vi "subGenPhaseContSine.vi"(0 "amplitude":dbl=1.0 format="%0.2p", 2 "reset signal":bool, 5 "frequency":dbl=10.0 format="%0.2p", 7 "phase":dbl format="%.2p", 11 "error in (no error)":errorcluster, 13 "sampling info":cluster{"Fs":dbl, "#s":dbl}={"Fs"=50000.0, "#s"=4000.0} {"Fs" format="%.2p"}) -> (4 "data":cluster{"t0":dbl, "dt":dbl, "Y":cdb[]}={"t0"=0.0, "dt"=1.0, "Y"=[]} {"Y" format="%.3f"; "dt" format="%^.2e"; "t0" format="%.4f"}, 8 "phase out":ext, 15 "error out":errorcluster)   [LabVIEW 2013]
uses:
  <vilib>/Analysis/1siggen.llb/Ramp Pattern by Samples.vi
  <vilib>/Analysis/NI_AALBase.lvlib
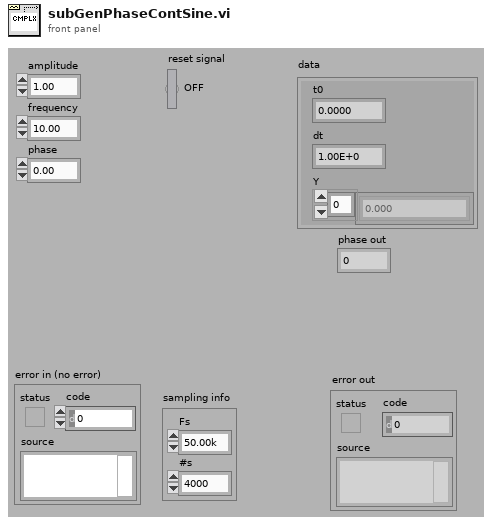
[diagram p1: front panel]
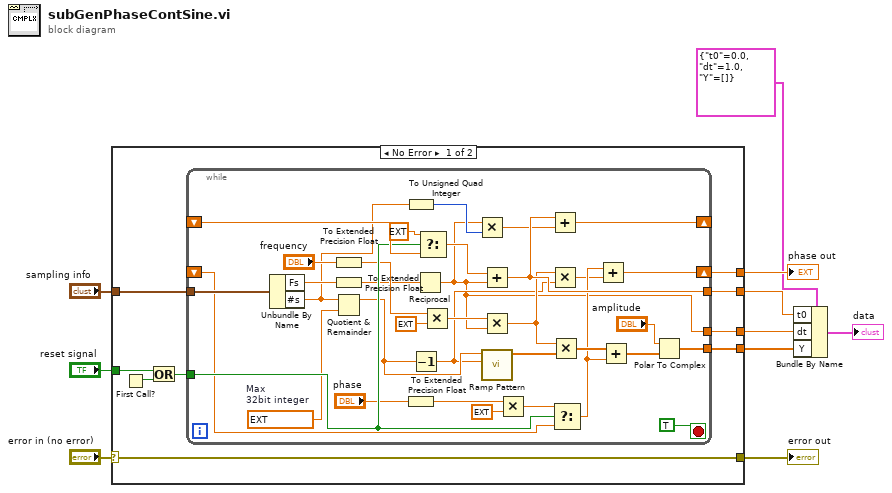
[diagram p0: block diagram]
diagram:
  n1 = case shown="No Error" "error in (no error)" {
    selector: "error in (no error)" -> [w11 w55]
    tunnel: "sampling info" -> [w19 _]
    tunnel: "reset signal" -> [w17 _]
    tunnel: [w11 w55] -> w8
    tunnel: [w15 _] -> w6
    tunnel: [w14 _] -> w5
    tunnel: [w13 _] -> w4
    tunnel: [w12 _] -> w3
    frame No Error {
      n2 = First Call?() -> (First Call?: T/F=w18:bool)
      n3 = Or(x=w17, y=w18) -> (x .or. y?=w16:bool)
      n4 = while {
        tunnel: w19 -> [w54]
        shift-right: [w44] -> w12
        shift-left: _ -> [w41]
        shift-right: [w50] -> _
        shift-left: _ -> [w49]
        tunnel: w16 -> [w42]
        tunnel: [w46] -> w15
        tunnel: [w20] -> w14
        tunnel: [w45] -> w13
        stop <- TRUE stop-if-true
        w30 = ext 2147483647.0  # Max  32bit integer
        n5 = Unbundle By Name(w54) -> ("Fs"=w51:dbl, "#s"=w23:dbl)
        n6 = To Extended Precision Float(1:"frequency") -> (0:w39:ext)
        n7 = To Extended Precision Float(1:w51) -> (0:w38:ext)
        n8 = Quotient & Remainder(x=w23, y=w30) -> (x-y*floor(x/y)=w24:ext)  [unwired: 1 out]
        n9 = To Unsigned Quad Integer(1:w23) -> (0:w29:u64)
        n10 = To Extended Precision Float(1:"phase") -> (0:w32:ext)
        n11 = Decrement(x=w24) -> (x-1=w21:ext)
        n12 = Reciprocal(x=w38) -> (1/x=w20:ext)
        n13 = Select(t=ext 0.0, s=w42, f=w49) -> (s? t:f=w48:ext)
        n14 = Multiply(x=w39, y=ext 6.283185307179586477) -> (x*y=w35:ext)
        n15 = Multiply(x=w20, y=w29) -> (x*y=w43:ext)
        n16 = Add(x=w48, y=w20) -> (x+y=w46:ext)
        n17 = Multiply(x=w35, y=w20) -> (x*y=w28:ext)
        n18 = call-poly <vilib>:"Ramp Pattern.vi"("end"=w21, "samples"=w24) -> ("Ramp Pattern"=w22:dbl[])  [unwired: 8 in, 1 out]
        n19 = Multiply(x=w32, y=ext 6.283185307179586477) -> (x*y=w31:ext)
        n20 = Add(x=w46, y=w43) -> (x+y=w50:ext)
        n21 = Multiply(x=w28, y=w21) -> (x*y=w26:ext)
        n22 = Multiply(x=w28, y=w22) -> (x*y=w37:ext[])
        n23 = Select(t=w31, s=w42, f=w41) -> (s? t:f=w27:ext)
        n24 = Add(x=w27, y=w26) -> (x+y=w44:ext)
        n25 = Add(x=w37, y=w27) -> (x+y=w36:ext[])
        n26 = Polar To Complex(1:w36, 2:"amplitude") -> (0:w45:cxt[])
      }
    }
    frame Error {
    }
  }
  "error out" <- w8
  "phase out" <- w3
  n27 = Bundle By Name(cluster=cluster{"t0":dbl, "dt":dbl, "Y":cdb[]} {"t0"=0.0, "dt"=1.0, "Y"=[]} ("data"), "t0"=w6, "dt"=w5, "Y"=w4) -> (→"data":cluster{"t0":dbl, "dt":dbl, "Y":cdb[]})
